vi "Serial_Playground.vi"() -> ()   [LabVIEW 2022 SP3]
uses:
  <vilib>/Instr/_visa.llb/VISA Configure Serial Port (Instr).vi
panel:
  in  "Filename":path=path "C:/Users/jlurv/Desktop/test.lvm"
  in  "stop":bool
  in  "termination char\n(0xA = '\\n' = LF)":u8=10 format="%.0x"
  in  "Byte Count":u32
  in  "Baud Rate":u32=9600
  in  "Serial Port":refnum<visa-resource-name>
  out "Waveform Chart":dbl[][](graph)
  # "Configuration Options"
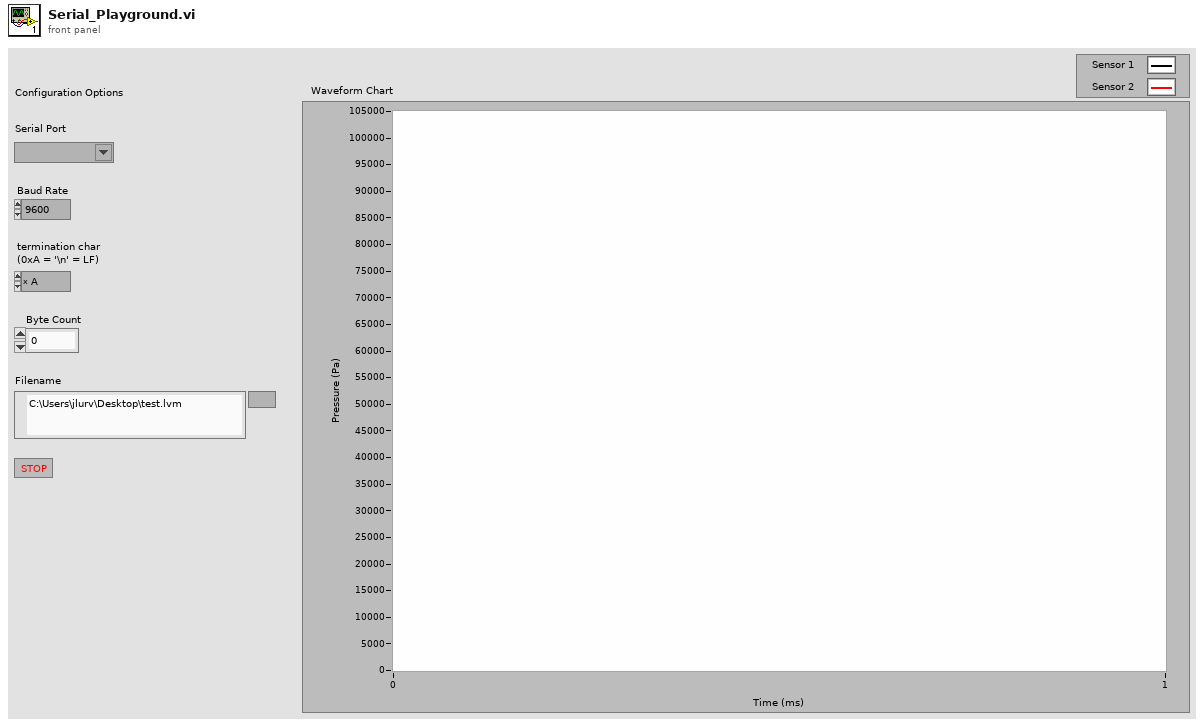
[diagram p1: front panel]
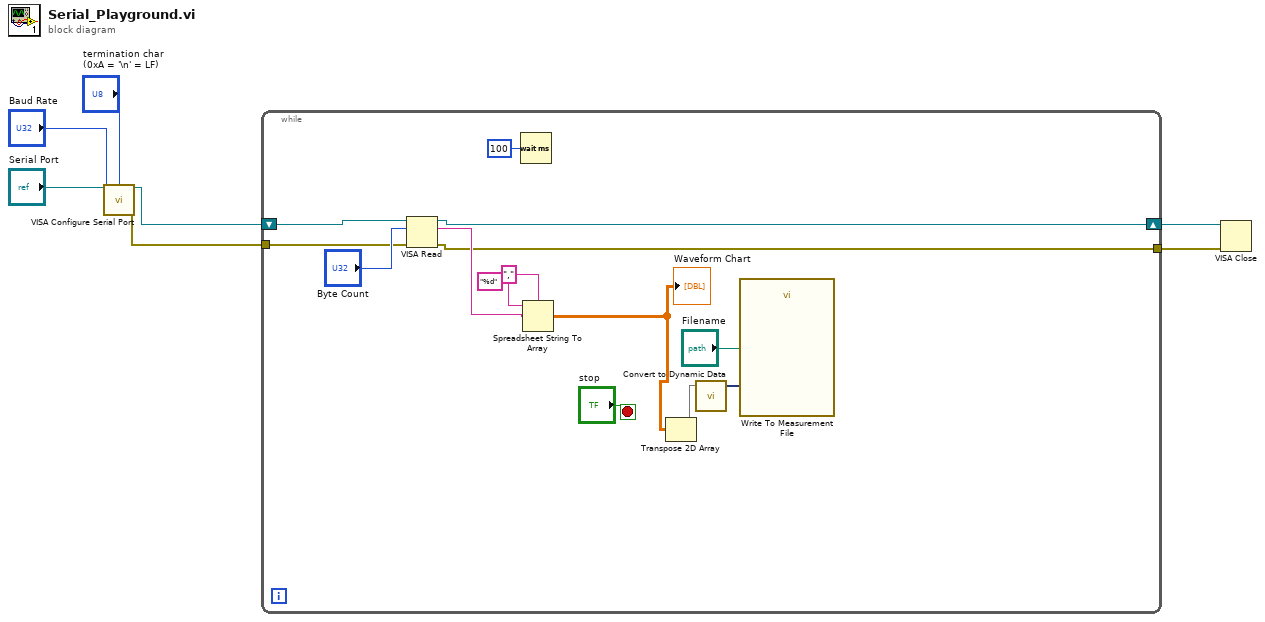
[diagram p0: block diagram]
diagram:
  n1 = call-poly "VISA Configure Serial Port"("VISA resource name"="Serial Port", "termination char\n(0xA = '\\n' = LF)"="termination char\n(0xA = '\\n' = LF)", "baud rate (9600)"="Baud Rate") -> ("VISA resource name out"=w5:refnum<visa-resource-name>, "error out"=w2:errorcluster)  [unwired: 11 in]
  n2 = while {
    shift-right: [w20] -> w4
    shift-left: w5 -> [w21]
    tunnel: w2 -> [w13]
    tunnel: [w12] -> w1
    stop <- "stop" stop-if-true
    n3 = VISA Read(VISA resource name=w21, byte count="Byte Count", error in (no error)=w13) -> (VISA resource name out=w20:refnum<visa-resource-name>, read buffer=w16:string, error out=w12:errorcluster)  [unwired: 1 out]
    n4 = Wait (ms)(milliseconds to wait=u32 100) -> ()  [unwired: 1 out]
    n5 = Spreadsheet String To Array(delimiter (Tab)=",", format string="%d", spreadsheet string=w16) -> (array=w10:dbl[][])  [unwired: 1 in]
    "Waveform Chart" <- w10
    n6 = Transpose 2D Array(2D array=w10) -> (transposed array=w9:dbl[][])
    n7 = call "Convert to Dynamic Data"("2D Array"=w9) -> ("Dynamic Data Type"=w11:dynamicdata)  [unwired: 3 in]
    n8 = call "Write To Measurement File"("Signals"=w11, "Filename"="Filename") -> ()  [unwired: 15 in, 3 out]
  }
  n9 = VISA Close(VISA resource name=w4, error in (no error)=w1) -> ()  [unwired: 1 out]
